vi "Create Folder.vi"(0 "Config File In":path, 11 "error in (no error)":errorcluster) -> (4 "Config File Out":path, 15 "error out":errorcluster)   [LabVIEW 2021, in "Packager Helpers.lvlib"]
uses:
  Packager Helpers.lvlib
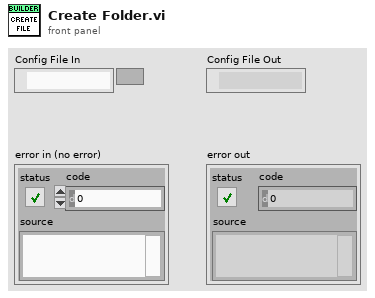
[diagram p1: front panel]
types:
  T1 = enum16{"open", "replace", "create", "open or create", "replace or create", "replace or create with confirmation"}
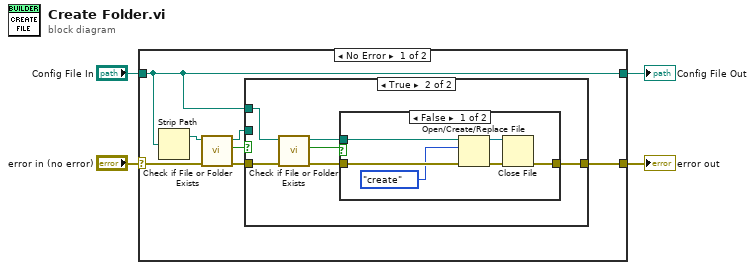
[diagram p0: block diagram]
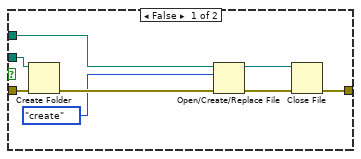
[diagram p2: hidden frame]
diagram:
  n1 = case shown="No Error" "error in (no error)" {
    selector: "error in (no error)" -> [w11 w34]
    tunnel: "Config File In" -> [w5 w33]
    tunnel: [w6 w34] -> w2
    tunnel: [w5 w33] -> w1
    frame No Error {
      n2 = Strip Path(path=w5) -> (stripped path=w10:path)  [unwired: 1 out]
      n3 = call <vilib>:"Check if File or Folder Exists.vi"("error in (no error)"=w11, "path"=w10) -> ("error out"=w9:errorcluster, "file or folder exists?"=w8:bool, "dup path"=w7:path)  [unwired: 7 in]
      n4 = case shown="True" w8 {
        tunnel: w9 -> [w19 w24]
        tunnel: w7 -> [w18 _]
        tunnel: [w12 w20] -> w6
        tunnel: w5 -> [w16 w25]
        frame False {
          n5 = Create Folder(path (use dialog)=w18, error in=w19) -> (error out=w17:errorcluster)  [unwired: 1 in, 2 out]
          n6 = Open/Create/Replace File(file path (use dialog)=w16, error in=w17, operation (0:open)=T1."create") -> (refnum out=w14:refnum<file>, error out=w13:errorcluster)  [unwired: 3 in, 1 out]
          n7 = Close File(refnum=w14, error in=w13) -> (error out=w12:errorcluster)  [unwired: 1 out]
        }
        frame True {
          n8 = call <vilib>:"Check if File or Folder Exists.vi"("error in (no error)"=w24, "path"=w25) -> ("error out"=w23:errorcluster, "file or folder exists?"=w22:bool, "dup path"=w21:path)  [unwired: 7 in]
          n9 = case shown="False" w22 {
            tunnel: w23 -> [w29 w32]
            tunnel: w21 -> [w28 _]
            tunnel: [w27 w32] -> w20
            frame False {
              n10 = Open/Create/Replace File(file path (use dialog)=w28, error in=w29, operation (0:open)=T1."create") -> (refnum out=w31:refnum<file>, error out=w30:errorcluster)  [unwired: 3 in, 1 out]
              n11 = Close File(refnum=w31, error in=w30) -> (error out=w27:errorcluster)  [unwired: 1 out]
            }
            frame True {
            }
          }
        }
      }
    }
    frame Error {
    }
  }
  "error out" <- w2
  "Config File Out" <- w1
